vi "Decimal Rounding Poly.vi"   [LabVIEW 2022 SP3]
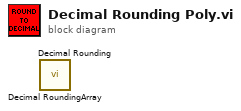
[diagram p0: block diagram]
diagram:
  n1 = call "Decimal RoundingArray.vi"() -> ()  [unwired: 11 in, 1 out]
  n2 = call "Decimal Rounding.vi"() -> ()  [unwired: 11 in, 1 out]
